vi "Raise Error for Sets Before 2024__ogtk.vi"(8 "error in (no error)":errorcluster) -> (0 "error out":errorcluster, 2 "supported?":bool)   [LabVIEW 2023, in "openg_variant.lvlib"]
uses:
  openg_variant.lvlib
  error/error.llb/openg_error.lvlib
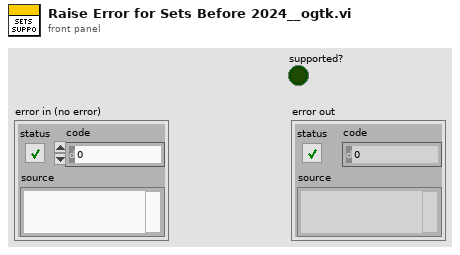
[diagram p1: front panel]
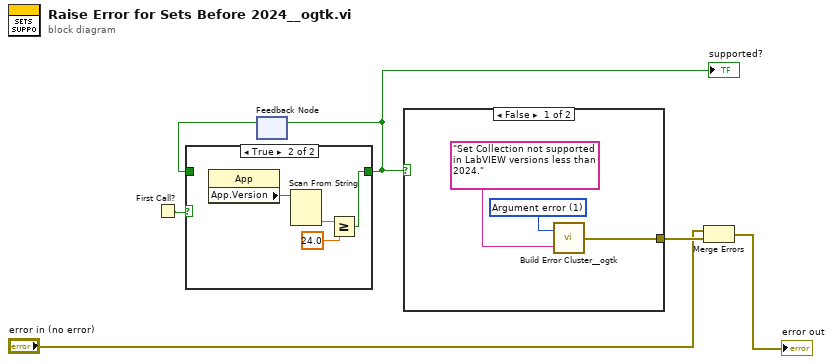
[diagram p0: block diagram]
diagram:
  n1 = First Call?() -> (First Call?: T/F=w3:bool)
  n2 = feedback #1() -> (w4:bool)  [unwired: 1 in]
  n3 = case shown="True" w3 {
    tunnel: w4 -> [w7 _]
    tunnel: [w7 w8] -> w5
    frame False {
    }
    frame True {
      n4 = property class="App"() -> ("App.Version"=w11:string)  [unwired: 2 in, 2 out]
      n5 = Scan From String(input string=w11) -> (output 1=w10:dbl)  [unwired: 4 in, 3 out]
      n6 = Greater Or Equal?(x=w10, y=24.0) -> (x >= y?=w8:bool)
    }
  }
  "supported?" <- w5
  n7 = feedback-in #1(w5) -> ()
  n8 = case shown="False" w5 {
    tunnel: [w12 _] -> w6
    frame False {
      w13 = 1 items=["No error", "Argument error", "Memory is full", "Out of zone", "End of file", "File already open", "Generic file I/O error", "File not found", "File permission error", "Disk is full", "Duplicate path", "Too many files open", "System feature not enabled", "Resource file not found", "Cannot add resource", "Resource not found", "Image not found", "Image memory error", "Pen does not exist", "Config type invalid", "Config token not found", "Config parse error", "Config memory error", "Bad external code format", "Bad external code offset", "External code not present", "Null window", "Destroy window error", "Null menu", "Print aborted", "Bad print record", "Print driver error", "Windows error during printing", "Memory error during printing", "Print dialog error", "Generic print error", "Invalid device refnum", "Device not found", "Device parameter error", "Device unit error", "Cannot open device", "Device call aborted", "Generic error", "Cancelled by user", "Object ID too low", "Object ID too high", "Object not in heap", "Unknown heap", "Unknown object (invalid DefProc)", "Unknown object (DefProc not in table)", "Message out of range", "Invalid (null) method", "Unknown message", "Manager call not supported", "Bad address", "Network operation in progress", "Network operation timed out", "Connection is busy", "Network attribute not supported", "Network error", "Address in use", "System out of memory", "Connection aborted", "Connection refused", "Not connected", "Already connected", "Connection closed", "Initialization error (interapplication manager)", "Bad occurrence", "Wait on unbound occurrence handler", "Occurrence queue overflow", "Datalog type conflict", "Unused", "Unrecognized type (interapplication manager)", "Memory corrupt", "Failed to make temporary DLL", "Old CIN version", "Drag socket not found", "Failed to load drop-object", "Failed to register OLE object", "Failed to release OLE object", "Format specifier type mismatch", "Unknown format specifier", "Too few format specifiers", "Too many format specifiers", "Scan failed", "Newer CIN version", "Error converting to variant", "Runtime menu error", "Password tampered", "Variant attribute not found", "Incompatible variant data type", "Event data is not available", "Event Store is not present", "Occurrence is not found", "Event Queue is not created", "Event info is not available", "Refnum passed is NULL", "Error retrieving Class GUID", "Error retrieving CoClass GUID", "Error retrieving TypeLib GUID.", "Bad built application magic bytes.", "Specific driver is different from the specific driver associated with the Logical Name.", "There is no session opened to the class driver.", "Max Error", "MAX - Error with config objects", "MAX - Error loading configuration", "MAX - Group not supported"]
      n9 = call "Build Error Cluster__ogtk.vi"("String to Prepend to source (\"\")"="Set Collection not supported in LabVIEW versions less than 2024." ("Format String"), "code"=w13) -> ("error out"=w12:errorcluster)
    }
    frame True {
    }
  }
  n10 = Merge Errors("error in (no error)", w6) -> (→"error out":errorcluster)
